vi "TEST - Get Last PString.vi"(8 "error in (no error)":errorcluster) -> (0 "error out":errorcluster, 2 "pass":bool)   [LabVIEW 2020]
uses:
  source/library/openg_variant.lvlib
panel:
  out "Failures":T1(array[cluster])
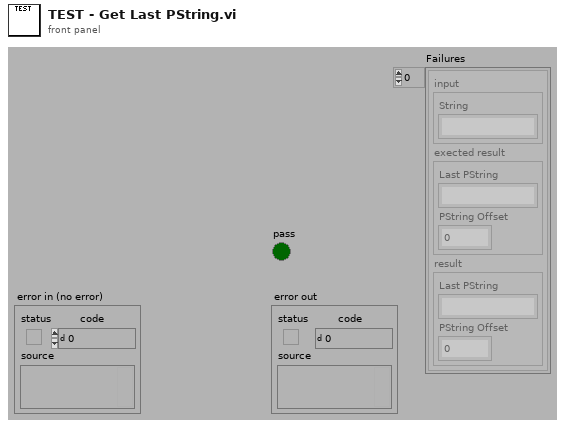
[diagram p1: front panel]
types:
  T1 = cluster{"input":cluster{"String":string}, "exected result":cluster{"Last PString":string, "PString Offset":i32}, "result":cluster{"Last PString":string, "PString Offset":i32}}[]
  T2 = cluster{"input":cluster{"String":string}, "exected result":cluster{"Last PString":string, "PString Offset":i32}, "result":cluster{"Last PString":string, "PString Offset":i32}}
  T3 = cluster{"Last PString":string, "PString Offset":i32}
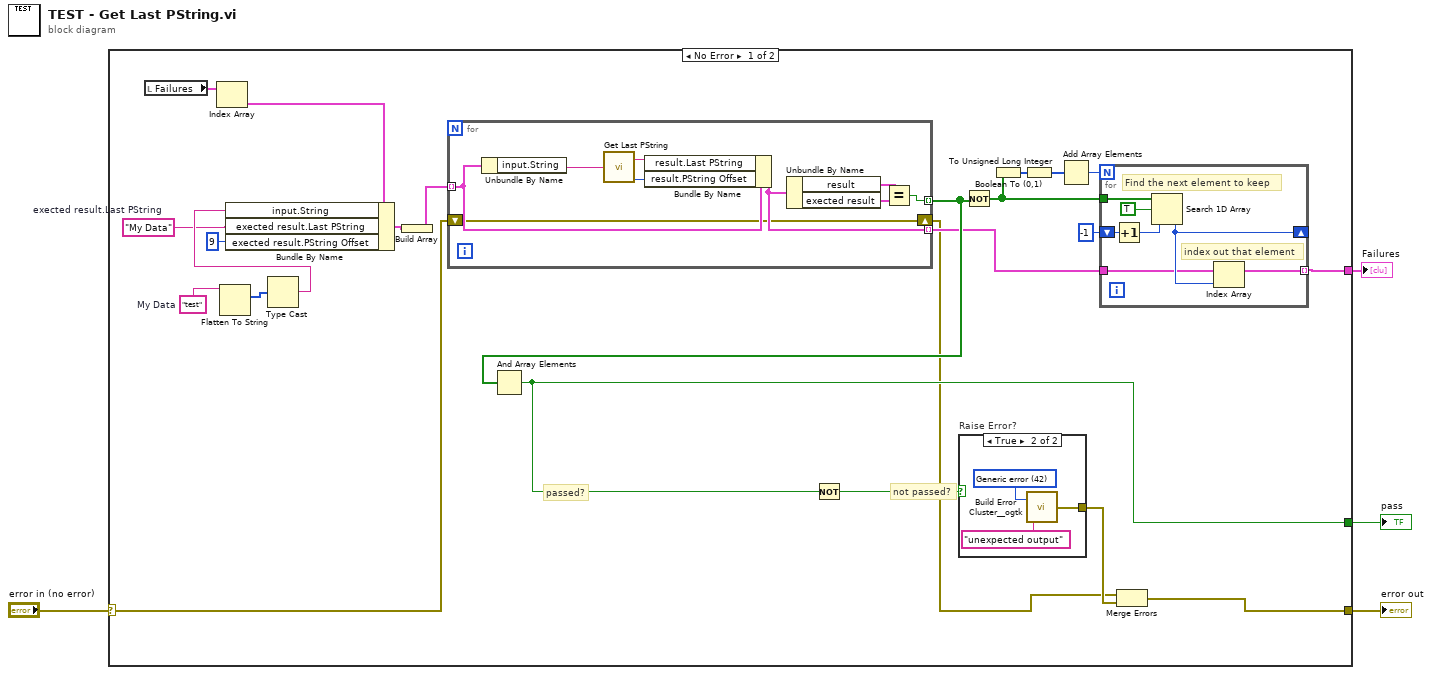
[diagram p0: block diagram]
diagram:
  n1 = case shown="No Error" "error in (no error)" {
    selector: "error in (no error)" -> [w13 w47]
    tunnel: [w24 _] -> w4
    tunnel: [w27 w47] -> w2
    tunnel: [w16 _] -> w1
    frame No Error {
      w5 = "My Data"  # exected result.Last PString
      w9 = "test"  # My Data
      # "not passed?"
      # "passed?"
      n2 = local read "Failures"() -> (w11:T1)
      n3 = Index Array(array=w11) -> (element=w10:T2)  [unwired: 1 in]
      n4 = Flatten To String(anything=w9) -> (type string=w8:i16[])  [unwired: 3 in, 2 out]
      n5 = Type Cast(x=w8) -> (*(type *) &x=w7:string)  [unwired: 1 in]
      n6 = Bundle By Name(cluster=w10, "input.String"=w7, "exected result.Last PString"=w5, "exected result.PString Offset"=9) -> (w15:T2)
      n7 = Build Array(w15) -> (w14:T1)
      n8 = for {
        tunnel: w14 -> [w42] mode=indexing
        tunnel: [w43] -> w18 mode=indexing
        tunnel: [w41] -> w17 mode=indexing
        shift-right: [w36] -> w12
        shift-left: w13 -> [w36]
        n9 = Unbundle By Name(w42) -> ("input.String"=w38:string)
        n10 = call "Get Last PString.vi"("String"=w38) -> ("Last PString"=w37:string, "PString Offset"=w35:i32)
        n11 = Bundle By Name(cluster=w42, "result.Last PString"=w37, "result.PString Offset"=w35) -> (w41:T2)
        n12 = Unbundle By Name(w41) -> ("result"=w40:T3, "exected result"=w39:T3)
        n13 = Equal?(x=w40, y=w39) -> (x = y?=w43:bool)
      }
      n14 = And Array Elements(Boolean array=w18) -> (logical AND=w24:bool)
      n15 = Not(x=w24) -> (.not. x?=w25:bool)
      n16 = case "Raise Error?" shown="True" w25 {
        tunnel: [_ w44] -> w26
        frame False {
        }
        frame True {
          w45 = 42 items=["No error", "Argument error", "Memory is full", "Out of zone", "End of file", "File already open", "Generic file I/O error", "File not found", "File permission error", "Disk is full", "Duplicate path", "Too many files open", "System feature not enabled", "Resource file not found", "Cannot add resource", "Resource not found", "Image not found", "Image memory error", "Pen does not exist", "Config type invalid", "Config token not found", "Config parse error", "Config memory error", "Bad external code format", "Bad external code offset", "External code not present", "Null window", "Destroy window error", "Null menu", "Print aborted", "Bad print record", "Print driver error", "Windows error during printing", "Memory error during printing", "Print dialog error", "Generic print error", "Invalid device refnum", "Device not found", "Device parameter error", "Device unit error", "Cannot open device", "Device call aborted", "Generic error", "Cancelled by user", "Object ID too low", "Object ID too high", "Object not in heap", "Unknown heap", "Unknown object (invalid DefProc)", "Unknown object (DefProc not in table)", "Message out of range", "Invalid (null) method", "Unknown message", "Manager call not supported", "Bad address", "Network operation in progress", "Network operation timed out", "Connection is busy", "Network attribute not supported", "Network error", "Address in use", "System out of memory", "Connection aborted", "Connection refused", "Not connected", "Already connected", "Connection closed", "Initialization error (interapplication manager)", "Bad occurrence", "Wait on unbound occurrence handler", "Occurrence queue overflow", "Datalog type conflict", "Unused", "Unrecognized type (interapplication manager)", "Memory corrupt", "Failed to make temporary DLL", "Old CIN version", "Drag socket not found", "Failed to load drop-object", "Failed to register OLE object", "Failed to release OLE object", "Format specifier type mismatch", "Unknown format specifier", "Too few format specifiers", "Too many format specifiers", "Scan failed", "Newer CIN version", "Error converting to variant", "Runtime menu error", "Password tampered", "Variant attribute not found", "Incompatible variant data type", "Event data is not available", "Event Store is not present", "Occurrence is not found", "Event Queue is not created", "Event info is not available", "Refnum passed is NULL", "Error retrieving Class GUID", "Error retrieving CoClass GUID", "Error retrieving TypeLib GUID.", "Bad built application magic bytes.", "Specific driver is different from the specific driver associated with the Logical Name.", "There is no session opened to the class driver.", "Max Error", "MAX - Error with config objects", "MAX - Error loading configuration", "MAX - Group not supported"]
          n17 = call <userlib>:"Build Error Cluster__ogtk.vi"("String to Prepend to source (\"\")"="unexpected output" ("String to Prepend to source (\"\")"), "code"=w45) -> ("error out"=w44:errorcluster)
        }
      }
      n18 = Not(x=w18) -> (.not. x?=w20:bool[])
      n19 = Boolean To (0,1)(Boolean=w20) -> (0, 1=w21:i16[])
      n20 = To Unsigned Long Integer(number=w21) -> (unsigned 32bit integer=w19:u32[])
      n21 = Add Array Elements(numeric array=w19) -> (sum=w22:u32)
      n22 = for {
        N: w22 -> [_]
        tunnel: w17 -> [w30]
        tunnel: w20 -> [w34]
        shift-right: [w31] -> _
        shift-left: -1 ("start index (0)") -> [w32]
        tunnel: [w29] -> w16 mode=indexing
        # "index out that element"
        # "Find the next element to keep"
        n23 = Increment(x=w32) -> (x+1=w28:i32)
        n24 = Search 1D Array(1D array=w34, element=TRUE, start index (0)=w28) -> (index of element=w31:i32)
        n25 = Index Array(array=w30, index=w31) -> (element=w29:T2)
      }
      n26 = Merge Errors(w12, w26) -> (w27:errorcluster)
    }
    frame Error {
    }
  }
  "pass" <- w4
  "error out" <- w2
  "Failures" <- w1
